vi "DDS_Clock.vi"() -> ()   [LabVIEW 2016] (continued)
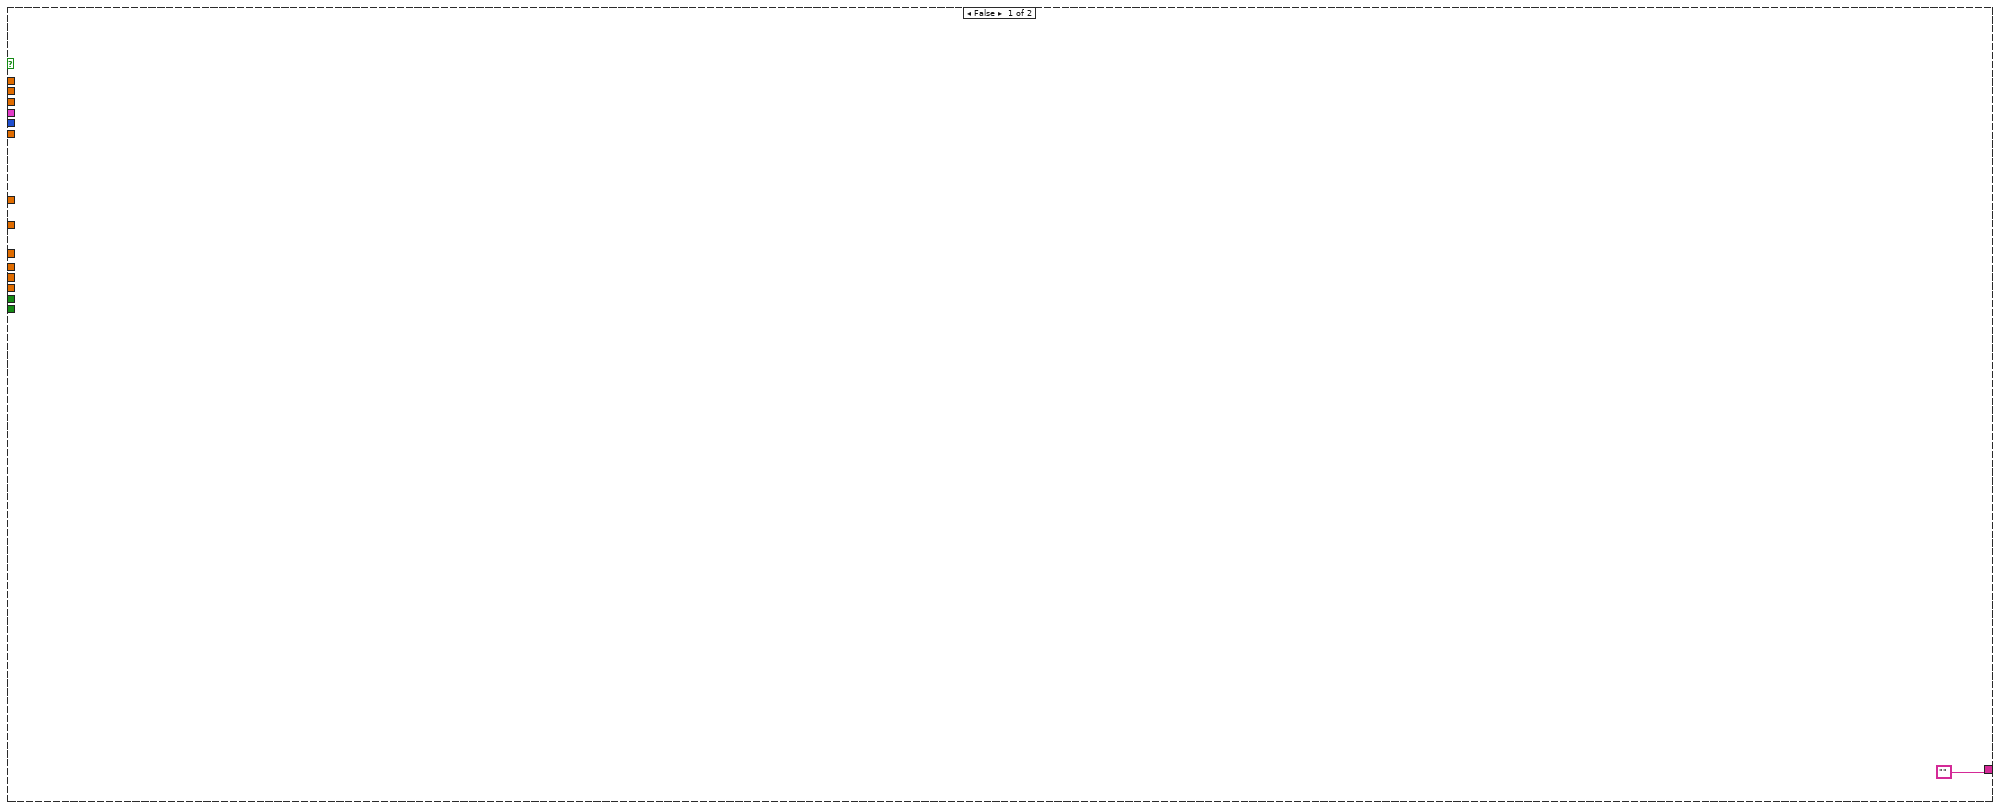
[diagram p2: hidden frame]
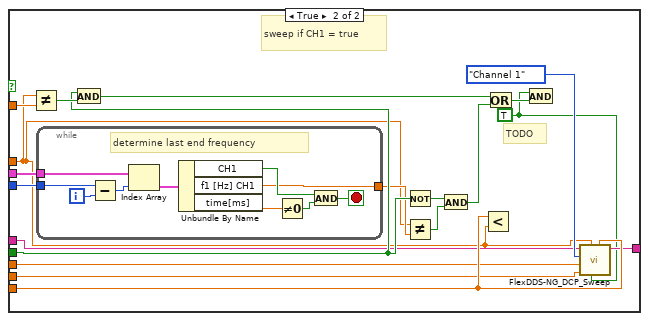
[diagram p3: hidden frame]
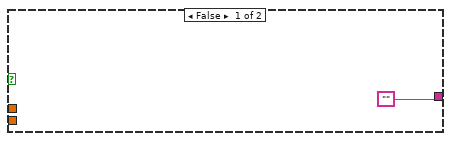
[diagram p6: hidden frame]
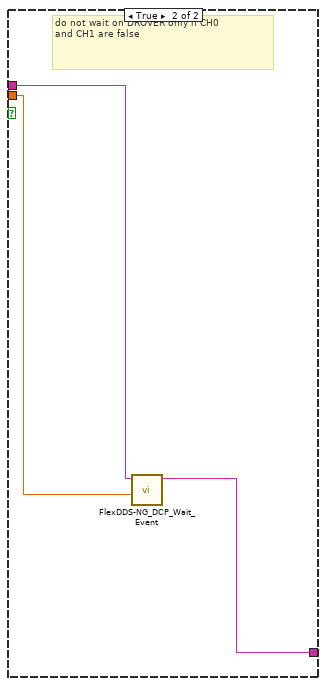
[diagram p7: hidden frame]
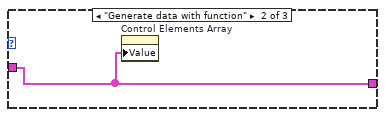
[diagram p8: hidden frame]
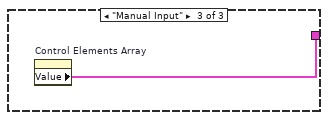
[diagram p9: hidden frame]
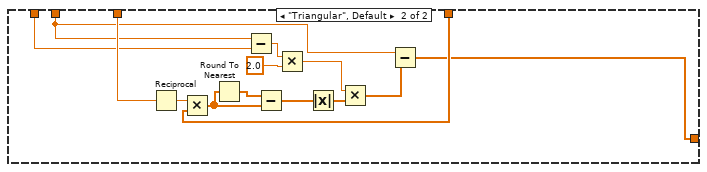
[diagram p14: hidden frame]
          n45 = property on="Control Elements Array" class="Arr (strict)"("Value"=w124) -> ()  [unwired: 2 in, 2 out]
        }
        frame "Manual Input" {
          n46 = property on="Control Elements Array" class="Arr (strict)"() -> ("Value"=w125:T5)  [unwired: 2 in, 2 out]
        }
      }
    }
    frame #1 {
      # "save array/settings or don't save anything"
      n47 = case shown="\"Save settings\"" "Store data" {
        tunnel: w127 -> [w128 _]
        frame "Save settings" {
          n48 = Flatten To XML(anything=w128) -> (xml string=w130:string)
          n49 = call-poly <vilib>:"Write to XML File.vi"("XML Input"=w130, "XML File Path"="XML File Path WRITE") -> ()  [unwired: 7 in, 3 out]
        }
        frame "Don't save settings", Default {
        }
      }
    }
    frame #2 {
      w134 = 0.0  # total time[ms]
      # "plot frequency time plot AFTER reading"
      n50 = for {
        tunnel: w131 -> [w168] mode=indexing
        shift-right: [w167] -> _
        shift-left: w134 -> [w163]
        tunnel: w131 -> [w164]
        shift-right: [w142] -> w138
        shift-left: T14 [] ("Array") -> [w143]
        shift-right: [w140] -> w139
        shift-left: T13 [] ("Array") -> [w141]
        i -> [w165]
        # "iterate through linear ramps;\nif time==0: skip;\nif CHx==false: keep frequency;"
        n51 = flat-sequence {
          tunnel: w165 -> [w178]
          tunnel: w164 -> [w179]
          tunnel: [w180] -> w152
          tunnel: [w177] -> w151
          frame #0 {
            # "i: current index\nif CHx == false, look for largest index j<i with CHx=true (to determine which frequency to plot)"
            n52 = while {
              tunnel: w178 -> [w200]
              tunnel: w179 -> [w197]
              tunnel: [w195] -> w180
              i -> [w199]
              stop <- w193 stop-if-true
              n53 = Subtract(x=w200, y=w199) -> (x-y=w198:i32)
              n54 = Index Array(array=w197, index=w198) -> (element=w196:T15)
              n55 = Unbundle By Name(w196) -> ("f1 [Hz] CH0"=w195:dbl, "CH0"=w192:bool, "time[ms]"=w194:dbl)
              n56 = Not Equal To 0?(x=w194) -> (x != 0?=w191:bool)
              n57 = And(x=w192, y=w191) -> (x .and. y?=w193:bool)
            }
            n58 = while {
              tunnel: w178 -> [w190]
              tunnel: w179 -> [w187]
              tunnel: [w185] -> w177
              i -> [w189]
              stop <- w183 stop-if-true
              n59 = Subtract(x=w190, y=w189) -> (x-y=w188:i32)
              n60 = Index Array(array=w187, index=w188) -> (element=w186:T15)
              n61 = Unbundle By Name(w186) -> ("f1 [Hz] CH1"=w185:dbl, "CH1"=w182:bool, "time[ms]"=w184:dbl)
              n62 = Not Equal To 0?(x=w184) -> (x != 0?=w181:bool)
              n63 = And(x=w182, y=w181) -> (x .and. y?=w183:bool)
            }
          }
        }
        n64 = Unbundle By Name(w168) -> ("time[ms]"=w166:dbl, "f0 [Hz] CH0"=w156:dbl, "f1 [Hz] CH0"=w155:dbl, "f0 [Hz] CH1"=w154:dbl, "f1 [Hz] CH1"=w153:dbl, "CH0"=w158:bool, "CH1"=w157:bool)
        n65 = Add(x=w163, y=w166) -> (x+y=w167:dbl)
        n66 = Not Equal To 0?(x=w166) -> (x != 0?=w144:bool)
        n67 = Select(t=w156, s=w158, f=w152) -> (s? t:f=w160:dbl)
        n68 = Select(t=w155, s=w158, f=w152) -> (s? t:f=w159:dbl)
        n69 = Select(t=w154, s=w157, f=w151) -> (s? t:f=w162:dbl)
        n70 = Select(t=w153, s=w157, f=w151) -> (s? t:f=w161:dbl)
        n71 = Bundle("total time[ms]"=w163, "f1 [Hz] CH0"=w160) -> (w150:cluster{"total time[ms]":dbl, "f1 [Hz] CH0":dbl})  [unwired: 1 in]
        n72 = Bundle(w167, "f1 [Hz] CH0"=w159) -> (w149:cluster{dbl, "f1 [Hz] CH0":dbl})  [unwired: 1 in]
        n73 = Bundle("total time[ms]"=w163, "f1 [Hz] CH1"=w162) -> (w148:cluster{"total time[ms]":dbl, "f1 [Hz] CH1":dbl})  [unwired: 1 in]
        n74 = Bundle(w167, "f1 [Hz] CH1"=w161) -> (w147:cluster{dbl, "f1 [Hz] CH1":dbl})  [unwired: 1 in]
        n75 = Build Array(w150, w149) -> (w146:T14)
        n76 = case shown="True" w144 {
          tunnel: w143 -> [w173 w175]
          tunnel: w146 -> [_ w174]
          tunnel: [w173 w176] -> w142
          frame False {
          }
          frame True {
            n77 = Build Array (concatenate)(w175, w174) -> (w176:T14)
          }
        }
        n78 = Build Array(w148, w147) -> (w145:T13)
        n79 = case shown="True" w144 {
          tunnel: w141 -> [w169 w171]
          tunnel: w145 -> [_ w170]
          tunnel: [w169 w172] -> w140
          frame False {
          }
          frame True {
            n80 = Build Array (concatenate)(w171, w170) -> (w172:T13)
          }
        }
      }
      n81 = Bundle("Array"=w138) -> (w135:T16)  [unwired: 1 in]
      n82 = Bundle("Array"=w139) -> (w136:T17)  [unwired: 1 in]
      n83 = Build Array(w135, w136) -> (→"frequency-time plot":T18)
    }
  }
  n84 = flat-sequence {
    frame #0 {
      # "This is the central data structure, work with property nodes to simplify reading and writing settings"
    }
  }
  n85 = flat-sequence {
    frame #0 {
      # "This is the central data structure, work with property nodes to simplify reading and writing settings"
    }
  }
  n86 = flat-sequence {
    tunnel: [w203] -> w19
    tunnel: [w201] -> w18
    tunnel: w12 -> [w201]
    tunnel: w19 -> [w209]
    tunnel: w18 -> [w204]
    tunnel: [w207] -> w17
    tunnel: [w204] -> w16
    tunnel: w17 -> [w212]
    tunnel: [w211] -> w15
    tunnel: w16 -> [w215]
    tunnel: [w215] -> w14
    tunnel: w15 -> [w216]
    tunnel: w14 -> [w220]
    tunnel: [w218] -> w13
    tunnel: [w447] -> w1
    tunnel: w13 -> [w446]
    frame #0 {
      # "Full Reset"
      n87 = call "FlexDDS-NG_DCP_Reset.vi"("full reset (yes)"=TRUE) -> ("appended instruction string"=w203:string)  [unwired: 10 in]
    }
    frame #1 {
      w208 = T19."Both channels" ("Channels")
      # "* inverse sinc filter\n* digital ramp enable\n* matched latency enable"
      # "Write CFR1 and CFR2"
      n88 = call "FlexDDS-NG_DCP_WriteCFR1_C.vi"("CFR1 bits"="CFR1 bits", "Channels"=w208, "initial instruction string"=w209) -> ("appended instruction string"=w210:string)  [unwired: 8 in]
      n89 = call "FlexDDS-NG_DCP_WriteCFR2_C.vi"("CFR2 bits"="CFR2 bits", "Channels"=w208, "initial instruction string"=w210) -> ("appended instruction string"=w207:string)  [unwired: 8 in]
    }
    frame #2 {
      # "add trigger"
      n90 = call "FlexDDS-NG_DCP_Wait_BNC.vi"("Trigger"="Wait for Trigger?", "Channels"=T19."Both channels" ("Channels 2"), "appended instruction string in"=w212) -> ("appended instruction string"=w211:string)  [unwired: 8 in]
    }
    frame #3 {
      # "iterate through array of clusters and create command string\nif 1st command is decreasing ramp add very short increasing ramp before\nignore all columns with time=0ms\nTODO: write some detailed documentation what is going on below"
      n91 = Array Size(array=w220) -> (size(s)=w221:i32)
      n92 = for {
        N: w221 -> [_]
        tunnel: w220 -> [w251] mode=indexing
        tunnel: w220 -> [w237]
        tunnel: [w250] -> w219 mode=indexing
        i -> [w249]
        # "iterate through array of time steps"
        n93 = Unbundle(w251) -> ("time[ms]"=w243:dbl, "time tolerance[us]"=w242:dbl, "CH0"=w248:bool, "rel. amplitude CH0"=w241:dbl, "phase [°] CH0"=w240:dbl, "f0 [Hz] CH0"=w247:dbl, "f1 [Hz] CH0"=w246:dbl, "CH1"=w222:bool, "rel. amplitude CH1"=w239:dbl, "phase [°] CH1"=w238:dbl, "f0 [Hz] CH1"=w245:dbl, "f1 [Hz] CH1"=w244:dbl)  [unwired: 1 out]
        n94 = flat-sequence {
          tunnel: w237 -> [w299]
          tunnel: w238 -> [w263]
          tunnel: w239 -> [w264]
          tunnel: w240 -> [w267]
          tunnel: w241 -> [w268]
          tunnel: w242 -> [w300]
          tunnel: w243 -> [w254]
          tunnel: w244 -> [w261]
          tunnel: w245 -> [w262]
          tunnel: w246 -> [w265]
          tunnel: w247 -> [w266]
          tunnel: w248 -> [w272]
          tunnel: w249 -> [w259]
          tunnel: [w259] -> w236
          tunnel: [w272] -> w235
          tunnel: [w269] -> w234
          tunnel: [w266] -> w233
          tunnel: [w265] -> w232
          tunnel: [w262] -> w231
          tunnel: [w261] -> w230
          tunnel: [w254] -> w229
          tunnel: [w300] -> w228
          tunnel: [w268] -> w227
          tunnel: [w267] -> w226
          tunnel: [w264] -> w225
          tunnel: [w263] -> w224
          tunnel: [w299] -> w223
          tunnel: w222 -> [w269]
          tunnel: [w315] -> w250
          tunnel: w236 -> [w314]
          tunnel: w235 -> [w313]
          tunnel: w234 -> [w312]
          tunnel: w233 -> [w302]
          tunnel: w232 -> [w301]
          tunnel: w231 -> [w311]
          tunnel: w230 -> [w310]
          tunnel: w229 -> [w309]
          tunnel: w228 -> [w303]
          tunnel: w227 -> [w308]
          tunnel: w226 -> [w307]
          tunnel: w225 -> [w306]
          tunnel: w224 -> [w305]
          tunnel: w223 -> [w304]
          frame #0 {
            # "0<=ampl<=1\n0<=freq<=400MHz\n0<=phase=360\nChx[0] not FALSE\ntime[0] not 0"
            # "check if input is valid\nabort otherwise"
            n95 = Equal To 0?(x=w259) -> (x = 0?=w256:bool)
            n96 = Equal To 0?(x=w254) -> (x = 0?=w255:bool)
            n97 = In Range and Coerce(upper limit=360.0, x=w267, lower limit=0.0) -> (In Range?=w279:bool)  [unwired: 1 out]
            n98 = In Range and Coerce(upper limit=360.0, x=w263, lower limit=0.0) -> (In Range?=w278:bool)  [unwired: 1 out]
            n99 = And(x=w256, y=w255) -> (x .and. y?=w253:bool)
            n100 = Not(x=w253) -> (.not. x?=w252:bool)
            n101 = Select(t=w272, s=w256, f=TRUE) -> (s? t:f=w274:bool)
            n102 = Select(t=w269, s=w256, f=TRUE) -> (s? t:f=w270:bool)
            n103 = In Range and Coerce(upper limit=400000000.0, x=w266, lower limit=0.0) -> (In Range?=w283:bool)  [unwired: 1 out]
            n104 = In Range and Coerce(upper limit=400000000.0, x=w265, lower limit=0.0) -> (In Range?=w282:bool)  [unwired: 1 out]
            n105 = In Range and Coerce(upper limit=400000000.0, x=w262, lower limit=0.0) -> (In Range?=w281:bool)  [unwired: 1 out]
            n106 = In Range and Coerce(upper limit=400000000.0, x=w261, lower limit=0.0) -> (In Range?=w280:bool)  [unwired: 1 out]
            n107 = In Range and Coerce(upper limit=1.0, x=w268, lower limit=0.0) -> (In Range?=w277:bool)  [unwired: 1 out]
            n108 = In Range and Coerce(upper limit=1.0, x=w264, lower limit=0.0) -> (In Range?=w276:bool)  [unwired: 1 out]
            n109 = Compound Arithmetic op=AND(w283, w282, w281, w280, w279, w278, w277, w276, w274, w270, w252) -> (w260:bool)
            n110 = Not(x=w260) -> (.not. x?=w258:bool)
            n111 = call "Display Message to User"("Enable"=w258) -> ("OK"=w257:bool)  [unwired: 9 in, 1 out]
            n112 = Stop(stop? (T)=w257) -> ()
          }
          frame #1 {
            n113 = Not Equal?(x=0.0, y=w309) -> (x != y?=w316:bool)
            n114 = case shown="True" w316 {
              tunnel: ["" w360] -> w315
              tunnel: w314 -> [_ w326]
              tunnel: w313 -> [_ w337]
              tunnel: w312 -> [_ w329]
              tunnel: w309 -> [_ w321]
              tunnel: w311 -> [_ w328]
              tunnel: w310 -> [_ w319]
              tunnel: w308 -> [_ w341]
              tunnel: w307 -> [_ w349]
              tunnel: w306 -> [_ w348]
              tunnel: w305 -> [_ w347]
              tunnel: w304 -> [_ w327]
              tunnel: w303 -> [_ w320]
              tunnel: w302 -> [_ w334]
              tunnel: w301 -> [_ w333]
              frame False {
              }
              frame True {
                # "1st iteration and amplitude or phase changed"
                # "skip if time is zero"
                n115 = Decrement(x=w326) -> (x-1=w359:i32)
                n116 = Not(x=w337) -> (.not. x?=w362:bool)
                n117 = Not(x=w329) -> (.not. x?=w361:bool)
                n118 = And(x=w362, y=w361) -> (x .and. y?=w363:bool)
                n119 = Index Array(array=w327, index=w359) -> (element=w332:T15)
                n120 = Unbundle By Name(w332) -> ("rel. amplitude CH0"=w355:dbl, "phase [°] CH0"=w354:dbl, "rel. amplitude CH1"=w351:dbl, "phase [°] CH1"=w350:dbl)
                n121 = Unbundle By Name(w332) -> ("CH0"=w330:bool, "CH1"=w323:bool, "f1 [Hz] CH0"=w331:dbl, "f1 [Hz] CH1"=w322:dbl)
                n122 = Equal?(x=w341, y=w355) -> (x = y?=w356:bool)
                n123 = Equal?(x=w349, y=w354) -> (x = y?=w357:bool)
                n124 = Equal?(x=w351, y=w348) -> (x = y?=w353:bool)
                n125 = And(x=w356, y=w357) -> (x .and. y?=w345:bool)
                n126 = Not(x=w345) -> (.not. x?=w344:bool)
                n127 = Equal To 0?(x=w326) -> (x = 0?=w358:bool)
                n128 = Or(x=w358, y=w344) -> (x .or. y?=w338:bool)
                n129 = And(x=w337, y=w338) -> (x .and. y?=w335:bool)
                n130 = case shown="True" w335 {
                  tunnel: w341 -> [_ w434]
                  tunnel: w349 -> [_ w433]
                  tunnel: ["" w432] -> w346
                  frame False {
                  }
                  frame True {
                    # "CH0: write stp if (i==0 or ampl/phase changed) and CH0 = true"
                    n131 = call "FlexDDS-NG_DCP_WriteSTP.vi"("phase degrees (0..360)"=w433, "amplitude (0..1)"=w434, "Channels"=T19."Channel 0", "initial instruction string"="") -> ("appended instruction string"=w432:string)  [unwired: 7 in]
                  }
                }
                n132 = Equal?(x=w350, y=w347) -> (x = y?=w352:bool)
                n133 = And(x=w353, y=w352) -> (x .and. y?=w343:bool)
                n134 = Not(x=w343) -> (.not. x?=w342:bool)
                n135 = Or(x=w358, y=w342) -> (x .or. y?=w339:bool)
                n136 = And(x=w329, y=w339) -> (x .and. y?=w336:bool)
                n137 = case shown="True" w336 {
                  tunnel: [w424 w429] -> w340
                  tunnel: w348 -> [_ w427]
                  tunnel: w347 -> [_ w426]
                  tunnel: w346 -> [w424 w425]
                  frame False {
                  }
                  frame True {
                    # "CH1: write stp if (i==0 or ampl/phase changed) and CH1 = true"
                    n138 = call "FlexDDS-NG_DCP_WriteSTP.vi"("phase degrees (0..360)"=w426, "amplitude (0..1)"=w427, "Channels"=T19."Channel 1", "initial instruction string"=w425) -> ("appended instruction string"=w429:string)  [unwired: 7 in]
                  }
                }
                n139 = case shown="True" w337 {
                  tunnel: w340 -> [w394 w401]
                  tunnel: [w394 w400] -> w325
                  tunnel: w321 -> [_ w398]
                  tunnel: w320 -> [_ w397]
                  tunnel: w334 -> [_ w399]
                  tunnel: w333 -> [_ w395]
                  tunnel: w331 -> [_ w412]
                  tunnel: w330 -> [_ w407]
                  tunnel: w327 -> [_ w405]
                  tunnel: w326 -> [_ w404]
                  frame False {
                  }
                  frame True {
                    w396 = TRUE ("x")
                    # "sweep if CH0 = true"
                    n140 = Not Equal?(x=w399, y=w412) -> (x != y?=w410:bool)
                    n141 = while {
                      tunnel: w405 -> [w423]
                      tunnel: w404 -> [w422]
                      tunnel: [w415] -> w403
                      i -> [w414]
                      stop <- w416 stop-if-true
                      # "determine last end frequency"
                      n142 = Subtract(x=w422, y=w414) -> (x-y=w421:i32)
                      n143 = Index Array(array=w423, index=w421) -> (element=w420:T15)
                      n144 = Unbundle By Name(w420) -> ("CH0"=w417:bool, "f1 [Hz] CH0"=w415:dbl, "time[ms]"=w419:dbl)
                      n145 = Not Equal To 0?(x=w419) -> (x != 0?=w418:bool)
                      n146 = And(x=w417, y=w418) -> (x .and. y?=w416:bool)
                    }
                    n147 = And(x=w407, y=w410) -> (x .and. y?=w411:bool)
                    n148 = Not(x=w407) -> (.not. x?=w408:bool)
                    n149 = Not Equal?(x=w399, y=w403) -> (x != y?=w406:bool)
                    n150 = And(x=w408, y=w406) -> (x .and. y?=w409:bool)
                    n151 = Or(x=w411, y=w409) -> (x .or. y?=w413:bool)
                    n152 = Less?(x=w395, y=w399) -> ()  [unwired: 1 out]
                    n153 = And(x=w396, y=w413) -> ()  [unwired: 1 out]
                    n154 = call "FlexDDS-NG_DCP_Sweep.vi"("f1"=w395, "jump before ramp"=w396, "f0"=w399, "sweep time tolerance (us)"=w397, "sweep time (ms)"=w398, "Channels in"=T19."Channel 0", "initial instruction string"=w401) -> ("appended instruction string out"=w400:string)  [unwired: 4 in]
                  }
                }
                n155 = case shown="False" w329 {
                  tunnel: w325 -> [w364 w370]
                  tunnel: [w364 w369] -> w324
                  tunnel: w321 -> [_ w367]
                  tunnel: w320 -> [_ w366]
                  tunnel: w328 -> [_ w368]
                  tunnel: w319 -> [_ w371]
                  tunnel: w322 -> [_ w382]
                  tunnel: w323 -> [_ w377]
                  tunnel: w327 -> [_ w375]
                  tunnel: w326 -> [_ w374]
                  frame False {
                  }
                  frame True {
                    w365 = TRUE ("x")
                    # "TODO"
                    # "sweep if CH1 = true"
                    n156 = Not Equal?(x=w368, y=w382) -> (x != y?=w380:bool)
                    n157 = while {
                      tunnel: w375 -> [w393]
                      tunnel: w374 -> [w391]
                      tunnel: [w384] -> w373
                      i -> [w392]
                      stop <- w385 stop-if-true
                      # "determine last end frequency"
                      n158 = Subtract(x=w391, y=w392) -> (x-y=w390:i32)
                      n159 = Index Array(array=w393, index=w390) -> (element=w389:T15)
                      n160 = Unbundle By Name(w389) -> ("CH1"=w386:bool, "f1 [Hz] CH1"=w384:dbl, "time[ms]"=w388:dbl)
                      n161 = Not Equal To 0?(x=w388) -> (x != 0?=w387:bool)
                      n162 = And(x=w386, y=w387) -> (x .and. y?=w385:bool)
                    }
                    n163 = And(x=w377, y=w380) -> (x .and. y?=w381:bool)
                    n164 = Not(x=w377) -> (.not. x?=w378:bool)
                    n165 = Not Equal?(x=w368, y=w373) -> (x != y?=w376:bool)
                    n166 = And(x=w378, y=w376) -> (x .and. y?=w379:bool)
                    n167 = Less?(x=w371, y=w368) -> ()  [unwired: 1 out]
                    n168 = Or(x=w381, y=w379) -> (x .or. y?=w383:bool)
                    n169 = And(x=w365, y=w383) -> ()  [unwired: 1 out]
                    n170 = call "FlexDDS-NG_DCP_Sweep.vi"("f1"=w371, "jump before ramp"=w365, "f0"=w368, "sweep time tolerance (us)"=w366, "sweep time (ms)"=w367, "Channels in"=T19."Channel 1", "initial instruction string"=w370) -> ("appended instruction string out"=w369:string)  [unwired: 4 in]
                  }
                }
                n171 = case shown="False" w363 {
                  tunnel: [w437 w445] -> w360
                  tunnel: w321 -> [_ w444]
                  tunnel: w324 -> [w436 w443]
                  frame False {
                    # "wait on DROVER if one of the channels\nwait 8ns (1h) before waiting on DROVER"
                    n172 = call "FlexDDS-NG_DCP_Wait_Event.vi"("waiting time [ms]"=8e-06, "Channels in"=T19."Both channels", "appended instruction string in"=w436) -> ("appended instruction string"=w438:string)  [unwired: 8 in]
                    n173 = call "FlexDDS-NG_DCP_Wait_Event.vi"("Event 1"=T20."DROVER", "Channels in"=T19."Both channels", "appended instruction string in"=w438) -> ("appended instruction string"=w437:string)  [unwired: 8 in]
                  }
                  frame True {
                    # "do not wait on DROVER only if CH0\nand CH1 are false"
                    n174 = call "FlexDDS-NG_DCP_Wait_Event.vi"("waiting time [ms]"=w444, "appended instruction string in"=w443) -> ("appended instruction string"=w445:string)  [unwired: 9 in]
                  }
                }
              }
            }
          }
        }
      }
      n175 = Concatenate Strings(w219) -> (w217:string)
      n176 = Format Into String(initial string=w216, w217) -> (resulting string=w218:string)  [unwired: 2 in, 1 out]
    }
    frame #4 {
      # "start"
      n177 = call "FlexDDS-NG_DCP_StartStop.vi"("initial instruction string"=w446) -> ("appended instruction string"=w447:string)  [unwired: 10 in]
    }
  }
  n178 = call "FlexDDS-NG_USB_VISA_Open.vi"("FlexDDS-NG USB VISA resource name (COM)"="FlexDDS-NG USB VISA resource name (COM)") -> ("error out"=w4:errorcluster, "FlexDDS-NG USB VISA resource name out"=w6:refnum<visa-resource-name>)  [unwired: 9 in]
  n179 = VISA Write(VISA resource name=w6, write buffer=w1, error in (no error)=w4) -> (VISA resource name out=w7:refnum<visa-resource-name>, return count=→"return count":u32, error out=w3:errorcluster)
  n180 = VISA Read(VISA resource name=w7, byte count=u32 500, error in (no error)=w3) -> (VISA resource name out=w10:refnum<visa-resource-name>, read buffer=→"read buffer":string, error out=→"error out":errorcluster)  [unwired: 1 out]
  n181 = VISA Close(VISA resource name=w10) -> ()  [unwired: 1 in, 1 out]
  "appended instruction string 2" <- w1
